vi "Data-Preview.vi"(6 "delimiter (/)":string="/", 8 "error in":errorcluster, 9 "ParentStr":string, 11 "data":variant) -> (0 "error out":errorcluster, 2 "Array":string[][](array[string]), 3 "data(dup)":variant)   [LabVIEW 2019, in "lv-apt-json-file.lvlib"]
uses:
  lv-apt-json-file.lvlib
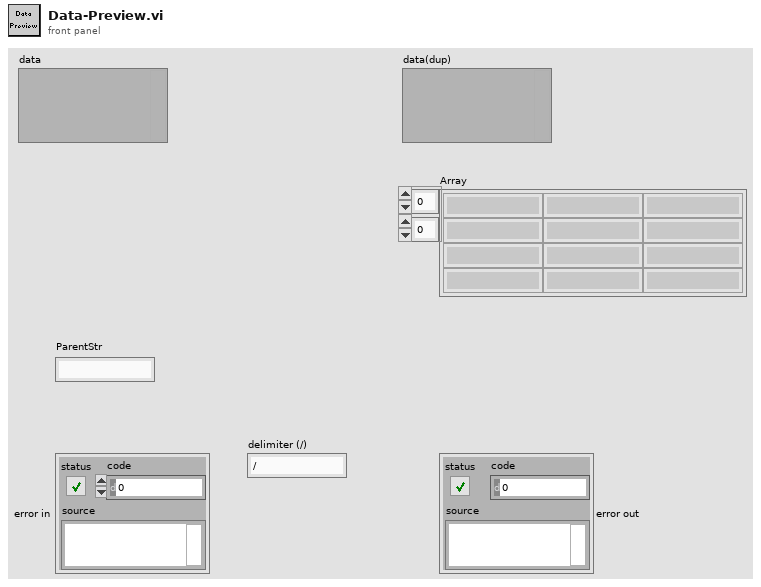
[diagram p1: front panel]
types:
  T1 = typedef "Type Descriptor Enumeration__ogtk.ctl" = enum8{"<Null>", "I8", "I16", "I32", "I64", "U8", "U16", "U32", "U64", "SGL", "DBL", "EXT", "CSG", "CDB", "CXT", "0x0F", "0x10", "0x11", "0x12", "0x13", "0x14", "Enum U8", "Enum U16", "Enum U32", "Enum U64", "SGL PQ", "DBL PQ", "EXT PQ", "CSG PQ", "CDB PQ", "CXT PQ", "0x1F", "0x20", "Boolean", "0x22", "0x23", "0x24", "0x25", "0x26", "0x27", "0x28", "0x29", "0x2A", "0x2B", "0x2C", "0x2D", "0x2E", "0x2F", "String", "0x31", "Path", "Pict", "0x34", "0x35", "0x36", "DAQ", "0x38", "0x39", "0x3A", "0x3B", "0x3C", "0x3D", "0x3E", "0x3F", "Array", "0x41", "0x42", "0x43", "0x44", "0x45", "0x46", "0x47", "0x48", "0x49", "0x4A", "0x4B", "0x4C", "0x4D", "0x4E", "0x4F", "Cluster", "0x51", "0x52", "Variant", "Waveform", "0x55", "0x56", "0x57", "0x58", "0x59", "0x5A", "0x5B", "0x5C", "0x5D", "0x5E", "0x5F", "0x60", "0x61", "0x62", "0x63", "0x64", "0x65", "0x66", "0x67", "0x68", "0x69", "0x6A", "0x6B", "0x6C", "0x6D", "0x6E", "0x6F", "Refnum"}
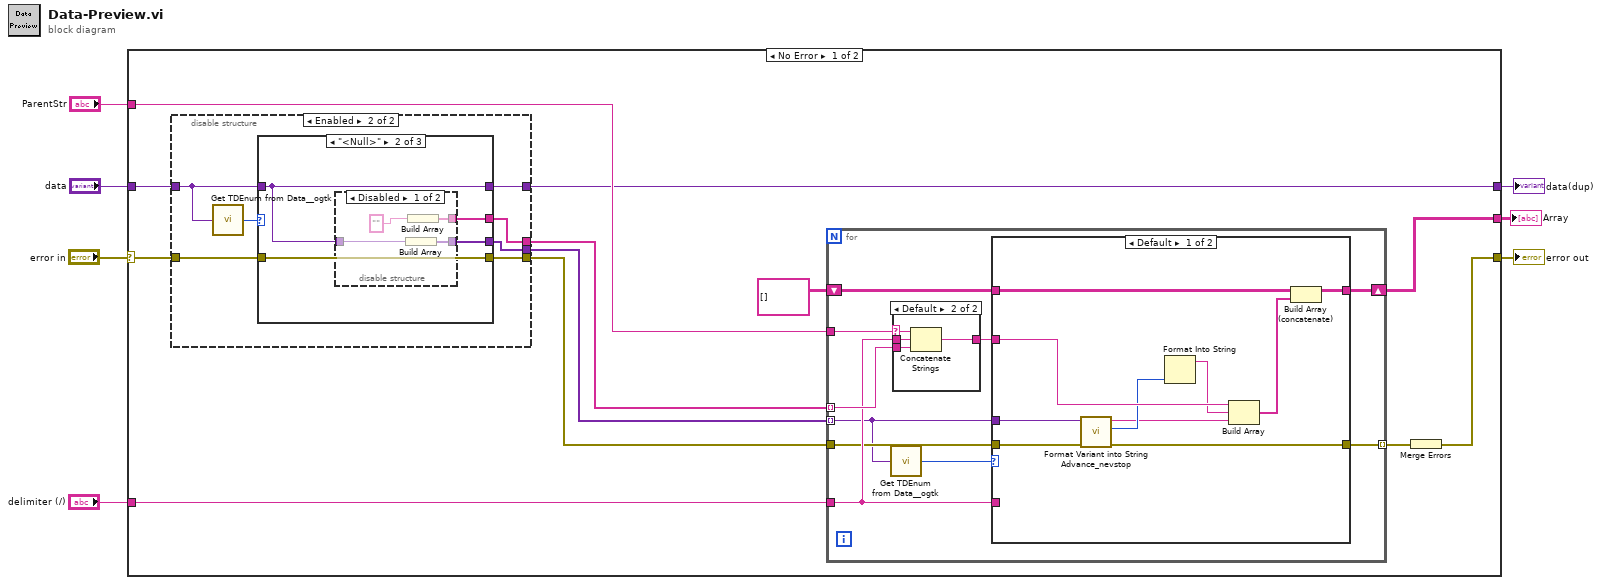
[diagram p0: block diagram]
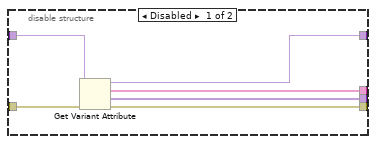
[diagram p2: hidden frame]
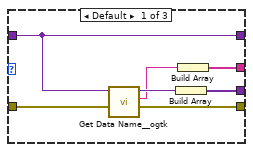
[diagram p3: hidden frame]
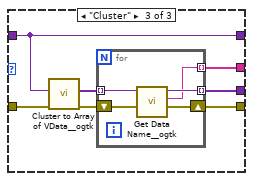
[diagram p5: hidden frame]
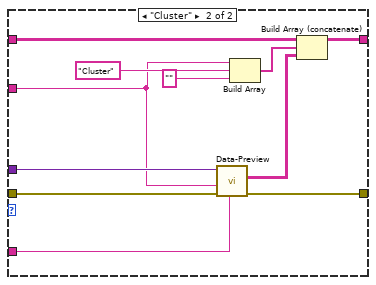
[diagram p7: hidden frame]
diagram:
  n1 = case shown="No Error" "error in" {
    selector: "error in" -> [w19 w97]
    tunnel: "data" -> [w10 w96]
    tunnel: [w9 w96] -> w5
    tunnel: [w12 w97] -> w4
    tunnel: [w16 _] -> w3
    tunnel: "ParentStr" -> [w15 _]
    tunnel: "delimiter (/)" -> [w11 _]
    frame No Error {
      n2 = disable-structure shown="Enabled" {
        disable-tunnel: w19 -> [w25 w29]
        disable-tunnel: [w24 w27] -> w18
        disable-tunnel: [w23 w26] -> w17
        disable-tunnel: w10 -> [w22 w30]
        disable-tunnel: [w21 w31] -> w9
        disable-tunnel: [w20 w28] -> w8
        frame Disabled {
          n3 = Get Variant Attribute(Variant=w22, error in=w25) -> (duplicate Variant=w21:variant, names=w23:string[], values=w24:variant[], error out=w20:errorcluster)  [unwired: 2 in]
        }
        frame Enabled {
          n4 = call <userlib>:"Get TDEnum from Data__ogtk.vi"("Data"=w30) -> ("Type Descriptor Enumeration"=w32:T1)  [unwired: 4 in]
          n5 = case shown="\"<Null>\"" w32 {
            tunnel: [w38 w42 w54] -> w31
            tunnel: w30 -> [w38 w42 w54]
            tunnel: w29 -> [w36 w41 w53]
            tunnel: [w35 w41 w49] -> w28
            tunnel: [w39 w43 w51] -> w27
            tunnel: [w33 w40 w48] -> w26
            frame Default {
              n6 = call <userlib>:"Get Data Name__ogtk.vi"("error in (no error)"=w36, "Data"=w38) -> ("error out"=w35:errorcluster, "Data Name"=w34:string, "Data dup"=w37:variant)  [unwired: 7 in]
              n7 = Build Array(w37) -> (w39:variant[])
              n8 = Build Array(w34) -> (w33:string[])
            }
            frame "<Null>" {
              n9 = disable-structure shown="Disabled" {
                disable-tunnel: [w47 _] -> w43
                disable-tunnel: w42 -> [w46 _]
                disable-tunnel: [w45 _] -> w40
                frame Disabled {
                  n10 = Build Array(w46) -> (w47:variant[])
                  n11 = Build Array("") -> (w45:string[])
                }
                frame Enabled {
                }
              }
            }
            frame "Cluster" {
              n12 = call <userlib>:"Cluster to Array of VData__ogtk.vi"("error in (no error)"=w53, "Cluster"=w54) -> ("error out"=w50:errorcluster, "Array of VData"=w52:variant[])  [unwired: 8 in]
              n13 = for {
                tunnel: w52 -> [w59] mode=indexing
                tunnel: [w58] -> w51 mode=indexing
                shift-right: [w56] -> w49
                shift-left: w50 -> [w57]
                tunnel: [w55] -> w48 mode=indexing
                n14 = call <userlib>:"Get Data Name__ogtk.vi"("error in (no error)"=w57, "Data"=w59) -> ("error out"=w56:errorcluster, "Data Name"=w55:string, "Data dup"=w58:variant)  [unwired: 7 in]
              }
            }
          }
        }
      }
      n15 = for {
        tunnel: w18 -> [w60] mode=indexing
        tunnel: w17 -> [w66] mode=indexing
        tunnel: w15 -> [w65]
        shift-right: [w67] -> w16
        shift-left: string[][] [] -> [w68]
        tunnel: w8 -> [w62]
        tunnel: [w69] -> w14 mode=indexing
        tunnel: w11 -> [w63]
        n16 = call <userlib>:"Get TDEnum from Data__ogtk.vi"("Data"=w60) -> ("Type Descriptor Enumeration"=w61:T1)  [unwired: 4 in]
        n17 = case shown="Default" w65 {
          selector: w65 -> [_ w73]
          tunnel: w66 -> [w70 w74]
          tunnel: [w70 w72] -> w64
          tunnel: w63 -> [_ w71]
          frame "" {
          }
          frame Default {
            n18 = Concatenate Strings(w73, w71, w74) -> (w72:string)
          }
        }
        n19 = case shown="Default" w61 {
          tunnel: w60 -> [w79 w86]
          tunnel: w62 -> [w78 w89]
          tunnel: [w77 w88] -> w69
          tunnel: w64 -> [w81 w85]
          tunnel: [w83 w94] -> w67
          tunnel: w68 -> [w84 w95]
          tunnel: w63 -> [_ w90]
          frame Default {
            n20 = call <userlib>:"Format Variant into String Advance_nevstop.vi"("error in (no error)"=w78, "Variant"=w79) -> ("error out"=w77:errorcluster, "Type Descriptor Enumeration"=w76:T1, "Data"=w75:string)  [unwired: 7 in]
            n21 = Format Into String(w76) -> (resulting string=w80:string)  [unwired: 3 in, 1 out]
            n22 = Build Array(w81, w80, w75) -> (w82:string[])
            n23 = Build Array (concatenate)(w84, w82) -> (w83:string[][])
          }
          frame "Cluster" {
            n24 = call "Data-Preview.vi"("delimiter (/)"=w90, "error in"=w89, "ParentStr"=w85, "data"=w86) -> ("error out"=w88:errorcluster, "Array"=w87:string[][])  [unwired: 5 in, 1 out]
            n25 = Build Array(w85, "Cluster" ("element"), "" ("element")) -> (w92:string[])
            n26 = Build Array (concatenate)(w95, w92, w87) -> (w94:string[][])
          }
        }
      }
      n27 = Merge Errors(w14) -> (w12:errorcluster)
    }
    frame Error {
    }
  }
  "error out" <- w4
  "data(dup)" <- w5
  "Array" <- w3
